vi "Create All Message Queues.vi"(8 "error in (no error)":errorcluster) -> (0 "error out":errorcluster, 3 "Message Queues out":T1)   [LabVIEW 2023, in "Weather Message Queue.lvlib"]
doc: "This VI creates and initializes all the message queues for the Weather Monitor application."
uses:
  Weather Message Queue.lvlib
  All Message Queues.ctl
  Message Cluster.ctl
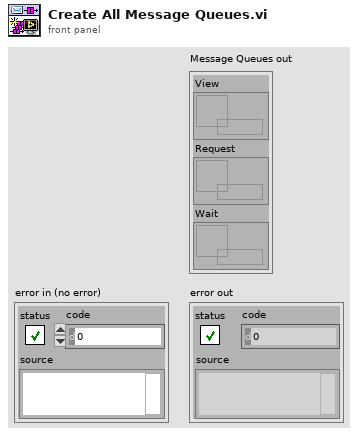
[diagram p1: front panel]
types:
  T1 = typedef "Weather Message Queue.lvlib/All Message Queues.ctl" = cluster{"View":refnum<queue>, "Request":refnum<queue>, "Wait":refnum<queue>}
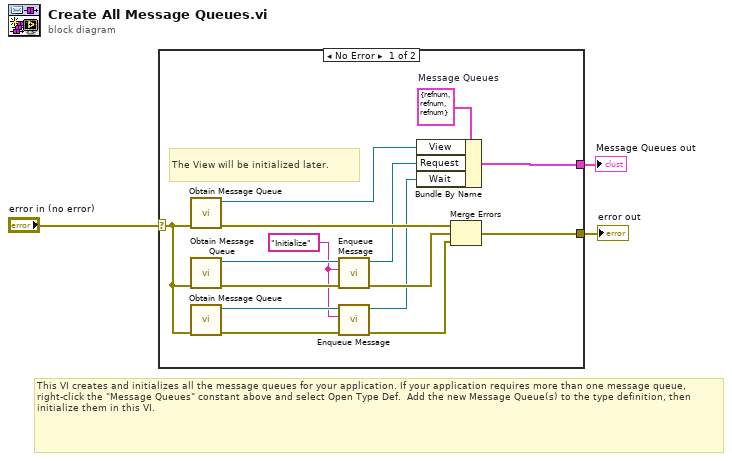
[diagram p0: block diagram]
diagram:
  # "This VI creates and initializes all the message queues for your application. If your application requires more than one message queue, right-click the \"Message Queues\" constant above and select Open Type Def.  Add the new Message Queue(s) to the type definition, then initialize them in this VI."
  n1 = case shown="No Error" "error in (no error)" {
    selector: "error in (no error)" -> [w7 w19]
    tunnel: [w11 w19] -> w3
    tunnel: [w17 _] -> w2
    frame No Error {
      w4 = "Initialize" ("Message")
      w18 = T1 {"View"=refnum, "Request"=refnum, "Wait"=refnum}  # Message Queues
      # "The View will be initialized later."
      n2 = call "Obtain Message Queue.vi"("error in (no error)"=w7) -> ("error out"=w16:errorcluster, "Message Queue"=w15:refnum<queue>)  [unwired: 9 in]
      n3 = call "Obtain Message Queue.vi"("error in (no error)"=w7) -> ("error out"=w13:errorcluster, "Message Queue"=w14:refnum<queue>)  [unwired: 9 in]
      n4 = call "Obtain Message Queue.vi"("error in (no error)"=w7) -> ("error out"=w9:errorcluster, "Message Queue"=w8:refnum<queue>)  [unwired: 9 in]
      n5 = call "Enqueue Message.vi"("error in (no error)"=w13, "Message"=w4, "Message Queue"=w14) -> ("error out"=w10:errorcluster, "dup Message Queue"=w12:refnum<queue>)  [unwired: 7 in]
      n6 = call "Enqueue Message.vi"("error in (no error)"=w9, "Message"=w4, "Message Queue"=w8) -> ("error out"=w6:errorcluster, "dup Message Queue"=w5:refnum<queue>)  [unwired: 7 in]
      n7 = Bundle By Name(cluster=w18, "View"=w15, "Request"=w12, "Wait"=w5) -> (w17:T1)
      n8 = Merge Errors(w16, w10, w6) -> (w11:errorcluster)
    }
    frame Error {
    }
  }
  "Message Queues out" <- w2
  "error out" <- w3
